vi "PH_PSDBWriter.add Data Status Service.vi"(0 "i ref in":refnum<vi>, 2 "Data Status":T1 items=["no info", "no Data collection", "no problem", "Error getting the ID", "Error writing Data", "Error getting the subsystem", "Error getting the Shot ID", "Error getting the Shot Types", "Error getting the Experiments", "Error verifying wanted Shottype", "Error verifying wanted Experiment"], 5 "error in (no error)":errorcluster) -> (14 "i ref out":refnum<vi>, 17 "Service ID Data Status":i32, 19 "error out":errorcluster)   [LabVIEW 2014, in "PH_PSDBWriter.lvlib"]
doc: "This VI publishes a status service \"<instancename>_Data_Status\", if no error comes in. For the status \n\n0: no info\n1: no Data collection\n2: no problem\n3: Error getting the Instance ID\n4: Error writing Data to data base\n\ncan be chosen. For further use, the Service ID is given out (it is \"-1\" if the service has not been added)."
uses:
  PH_PSDBWriter.lvlib
  PH_PSDBWriter.Data Status.ctl
  CSlibraries-extern/DimLVEvent/LVDimInterface/LVDimInterface.lvlib
  CS_Core/CSSystem/CSSystemLib/CSSystemLib.lvlib
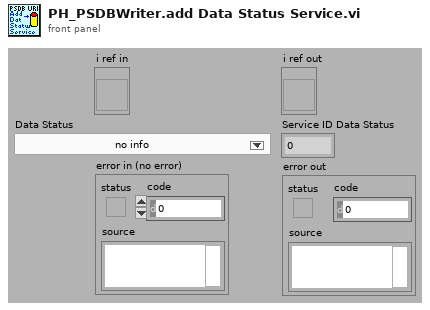
[diagram p1: front panel]
types:
  T1 = typedef "PH_PSDBWriter.lvlib/PH_PSDBWriter.Data Status.ctl" = i16
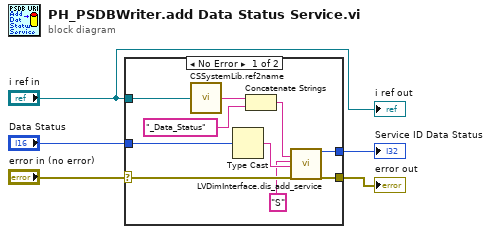
[diagram p0: block diagram]
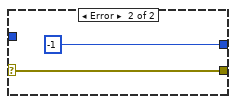
[diagram p2: hidden frame]
diagram:
  n1 = case shown="No Error" "error in (no error)" {
    selector: "error in (no error)" -> [w12 w17]
    tunnel: [w15 -1 ("my_serviceID")] -> w5
    tunnel: [w14 w17] -> w4
    tunnel: "Data Status" -> [w11 _]
    tunnel: "i ref in" -> [w13 _]
    frame No Error {
      n2 = call "CSSystemLib.ref2name.vi"("obj refnum"=w13) -> ("name"=w8:string)
      n3 = Type Cast(x=w11) -> (*(type *) &x=w10:string)  [unwired: 1 in]
      n4 = Concatenate Strings(w8, "_Data_Status" ("string")) -> (w7:string)
      n5 = call "LVDimInterface.dis_add_service.vi"("serviceName"=w7, "typeDescriptor"="S", "data"=w10, "error in (no error)"=w12) -> ("my_serviceID"=w15:i32, "error out"=w14:errorcluster)  [unwired: 14 in]
    }
    frame Error {
    }
  }
  "Service ID Data Status" <- w5
  "error out" <- w4
  "i ref out" <- "i ref in"
